vi "goto firmware.vi"(8 "error in (no error)":errorcluster, 10 "ret":u8, 11 "id":i32) -> (0 "error out":errorcluster, 2 "ret out":u8, 3 "function return":i32)   [LabVIEW 2012, in "libximc.lvlib"]
doc: "result_t XIMC_API goto_firmware(device_t id, uint8_t* ret);"
uses:
  libximc.lvlib
  libximc.dll
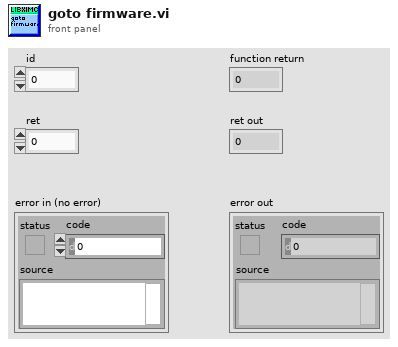
[diagram p1: front panel]
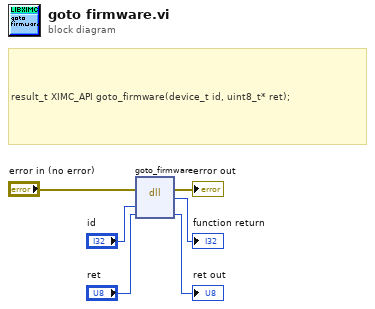
[diagram p0: block diagram]
diagram:
  # "result_t XIMC_API goto_firmware(device_t id, uint8_t* ret);"
  n1 = dll-call lib="C:/Users/Vasily/Att_examples/LabVIEW_example/libximc.*" fn="goto_firmware"(error in="error in (no error)", "id"="id", "ret"="ret") -> (error out=→"error out":errorcluster, →"function return":i32, "ret"=→"ret out":u8)  [unwired: 3 in, 1 out]
